vi "Plugin - Long Offset.vi"(11 "Message Queues in":T2) -> ()   [LabVIEW 2019]
uses:
  support/Copy of Message Queue/All Message Queues.ctl
  support/Copy of Message Queue/Message Cluster.ctl
  controls/WhieBackgroundHistogram.ctl
  Analysis/Global Tube Measurement.vi
  Acquisition/Acquisition.lvlib
  Analysis/Analysis.lvlib
  <vilib>/Analysis/NI_AALBase.lvlib
  <vilib>/ptbypt/NI_PtbyPt.lvlib
  support/Message Queue/Message Queue.lvlib
  support/Copy of Message Queue/Copy of Message Queue.lvlib
panel:
  out "Range(m)":dbl
  out "Ring Time (ms)":dbl format="%.2f"
  out "SSC Out(m)":dbl format="%0.4f"
  out "Offset Mean(m)":dbl format="%0.4f"
  out "Offset Std(m)":dbl format="%0.4f"
  in  "Stop":bool
  out "Time vs. Offset/Cor Offset":cluster{"Cor Offset":dbl, "Offset":dbl}(graph)
  out "Histogram Graph":T1
  out "T12":dbl(slide) scale=0.0..30.0
  out "T11":dbl(slide) scale=0.0..30.0
  out "T10":dbl(slide) scale=0.0..30.0
  out "T9":dbl(slide) scale=0.0..30.0
  out "T8":dbl(slide) scale=0.0..30.0
  out "T7":dbl(slide) scale=0.0..30.0
  out "T6":dbl(slide) scale=0.0..30.0
  out "T5":dbl(slide) scale=0.0..30.0
  out "T4":dbl(slide) scale=0.0..30.0
  out "T3":dbl(slide) scale=0.0..30.0
  out "T2":dbl(slide) scale=0.0..30.0
  out "T1":dbl(slide) scale=0.0..30.0
  out "Ring Time":waveform(dbl)(graph)
  out "Aquatrak RS232 Output":string
  in  "error in":errorcluster
  out "error out":errorcluster
  # "Calulating Long Offset"
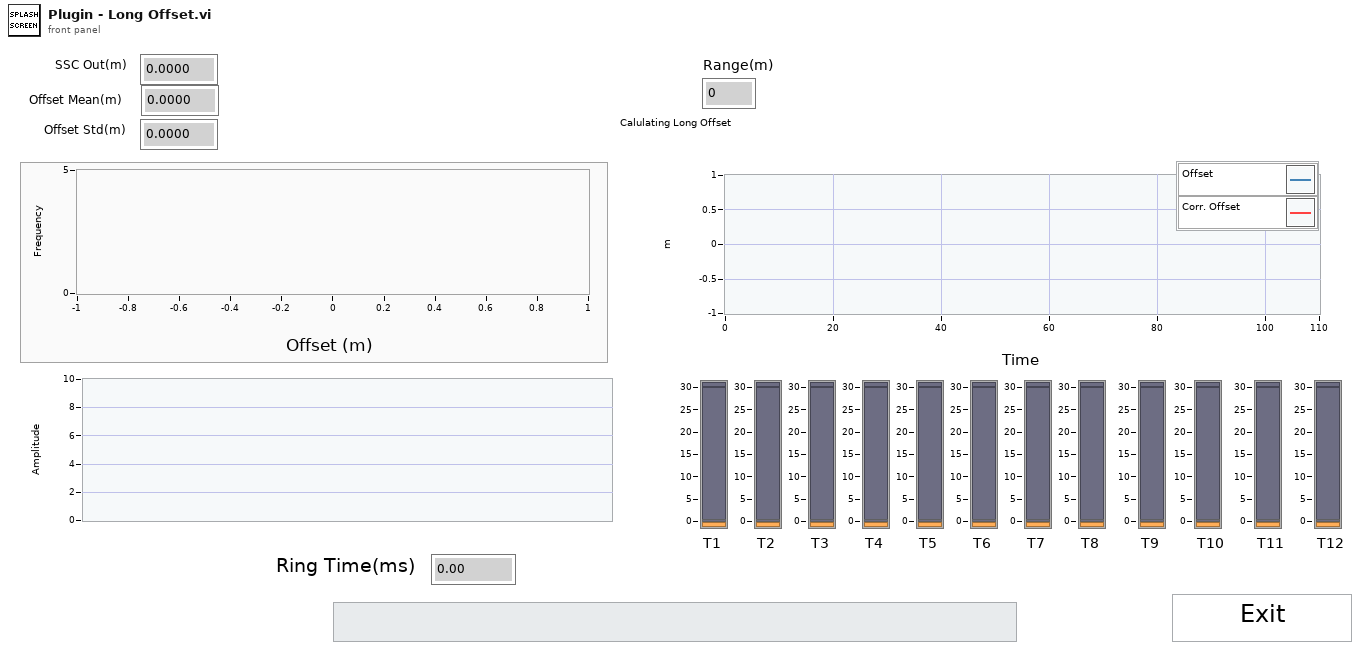
[diagram p1: front panel]
types:
  T1 = typedef "WhieBackgroundHistogram.ctl" = cluster{"X Values":dbl[], "Histogram: h(x)":i32[]}
  T2 = typedef "Copy of Message Queue.lvlib/All Message Queues.ctl" = cluster{"UI":refnum<queue>, "Acquisition":refnum<queue>, "Logging":refnum<queue>, "Analyze":refnum<queue>}
  T3 = cluster{"X Values":dbl[], "Histogram: h(x)":i32[]}
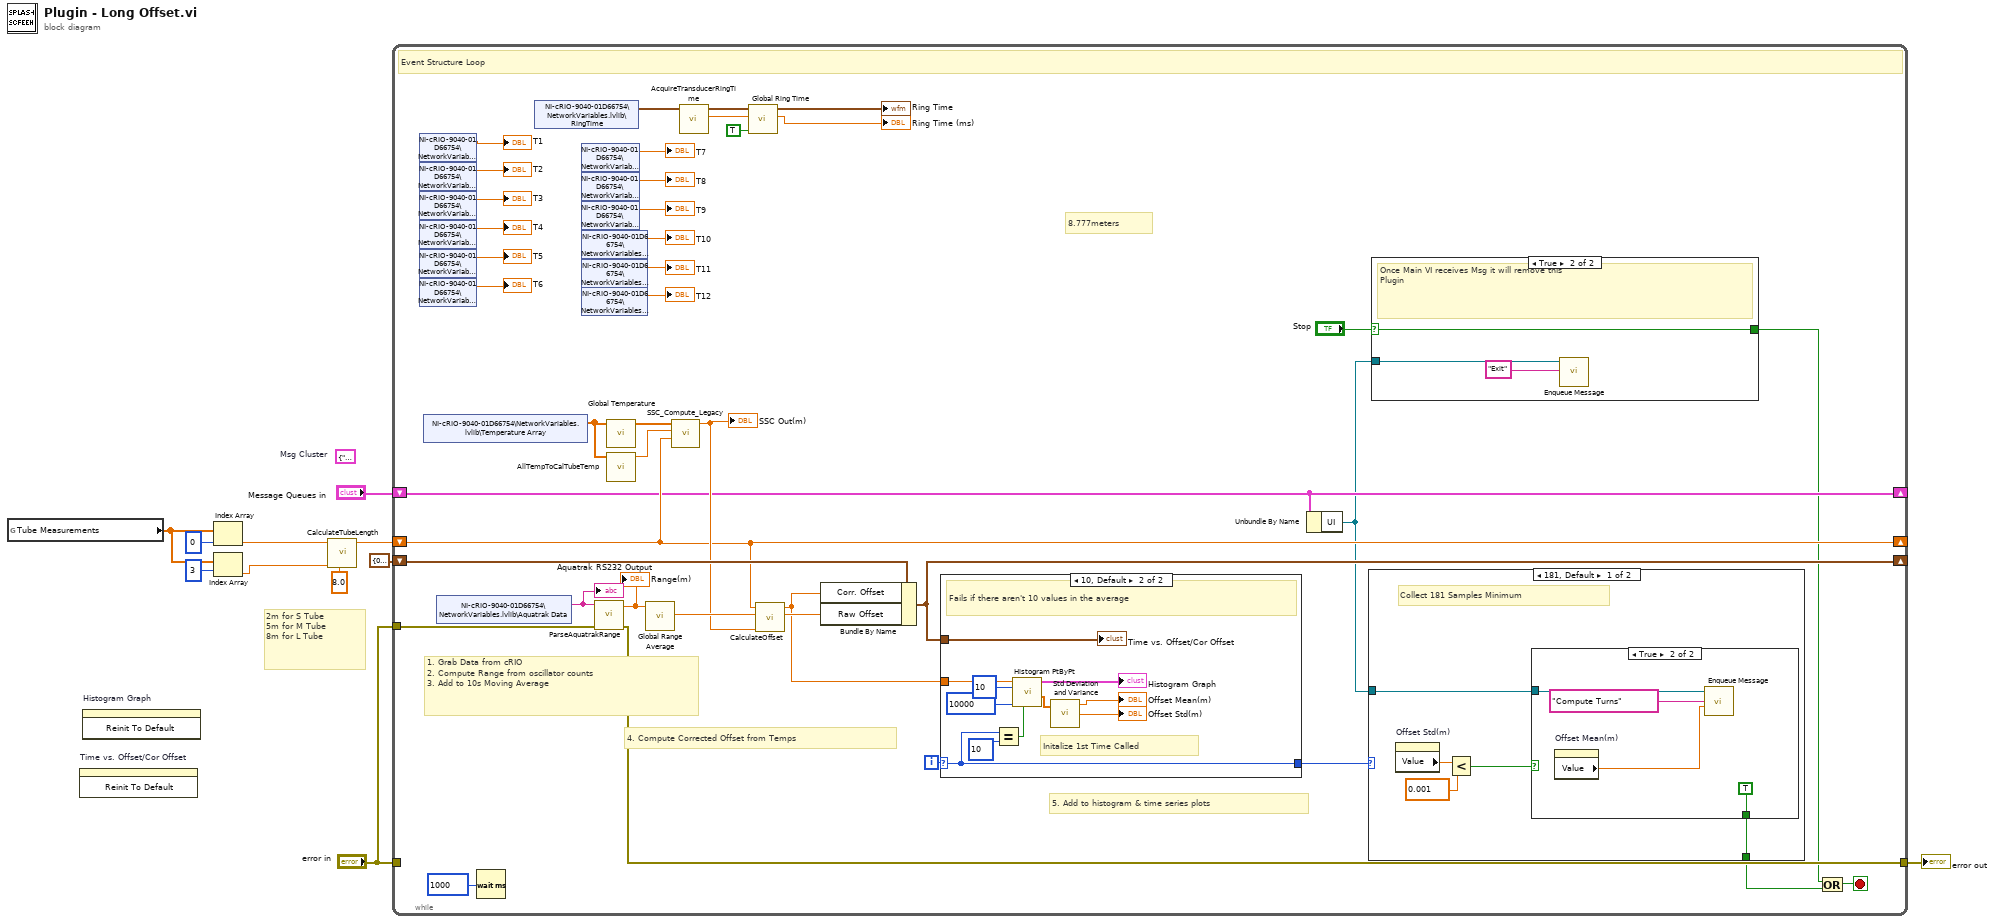
[diagram p0: block diagram]
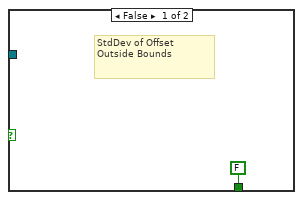
[diagram p3: hidden frame]
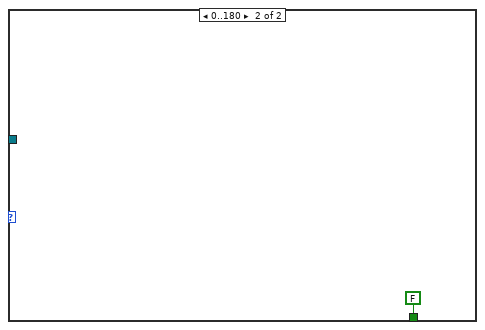
[diagram p4: hidden frame]
diagram:
  (unwired) cluster{"Msg":string, "Data":variant} {"Msg"="", "Data"=variant}  # Msg Cluster
  # "2m for S Tube\n5m for M Tube\n8m for L Tube"
  n1 = global read "Global Tube Measurement.vi" "Tube Measurements"() -> (w10:dbl[])
  n2 = invoke on="Time vs. Offset/Cor Offset" class="WFChart (strict)" method="Reinit To Default"() -> ()  [unwired: 3 in, 3 out]
  n3 = invoke on="Histogram Graph" class="XYGraph (strict)" method="Reinit To Default"() -> ()  [unwired: 3 in, 3 out]
  n4 = Index Array(array=w10, index=0) -> (element=w6:dbl)
  n5 = Index Array(array=w10, index=3) -> (element=w1:dbl)
  n6 = call "CalculateTubeLength.vi"("Range"=8.0, "Long Tube"=w1, "Collar"=w6) -> ("Tube Length"=w7:dbl)  [unwired: 8 in]
  n7 = while {
    shift-right: [w18] -> _
    shift-left: "Message Queues in" -> [w18]
    tunnel: "error in" -> [_]
    shift-right: [w20] -> _
    shift-left: cluster{"Raw Offset":dbl, "Corr. Offset":dbl} {"Raw Offset"=0.0, "Corr. Offset"=0.0} -> [w36]
    shift-right: [w21] -> _
    shift-left: w7 -> [w21]
    tunnel: [w25] -> w4
    tunnel: "error in" -> [w26]
    i -> [w22]
    stop <- w15 stop-if-true
    # "8.777meters"
    # "5. Add to histogram & time series plots"
    # "4. Compute Corrected Offset from Temps"
    # "1. Grab Data from cRIO\n2. Compute Range from oscillator counts \n3. Add to 10s Moving Average"
    # "Event Structure Loop"
    n8 = shared-variable "NI-cRIO-9040-01D66754\\NetworkVariables.lvlib\\T1"() -> (→"T1":dbl)  [unwired: 1 in, 1 out]
    n9 = shared-variable "NI-cRIO-9040-01D66754\\NetworkVariables.lvlib\\T2"() -> (→"T2":dbl)  [unwired: 1 in, 1 out]
    n10 = shared-variable "NI-cRIO-9040-01D66754\\NetworkVariables.lvlib\\T3"() -> (→"T3":dbl)  [unwired: 1 in, 1 out]
    n11 = shared-variable "NI-cRIO-9040-01D66754\\NetworkVariables.lvlib\\T4"() -> (→"T4":dbl)  [unwired: 1 in, 1 out]
    n12 = shared-variable "NI-cRIO-9040-01D66754\\NetworkVariables.lvlib\\T5"() -> (→"T5":dbl)  [unwired: 1 in, 1 out]
    n13 = shared-variable "NI-cRIO-9040-01D66754\\NetworkVariables.lvlib\\T6"() -> (→"T6":dbl)  [unwired: 1 in, 1 out]
    n14 = shared-variable "NI-cRIO-9040-01D66754\\NetworkVariables.lvlib\\Temperature Array"() -> (w34:dbl[])  [unwired: 1 in, 1 out]
    n15 = shared-variable "NI-cRIO-9040-01D66754\\NetworkVariables.lvlib\\Aquatrak Data"() -> (w35:string)  [unwired: 1 in, 1 out]
    "Aquatrak RS232 Output" <- w35
    n16 = Wait (ms)(milliseconds to wait=u32 1000) -> ()  [unwired: 1 out]
    n17 = shared-variable "NI-cRIO-9040-01D66754\\NetworkVariables.lvlib\\RingTime"() -> (w52:waveform(dbl)[])  [unwired: 1 in, 1 out]
    n18 = shared-variable "NI-cRIO-9040-01D66754\\NetworkVariables.lvlib\\T7"() -> (→"T7":dbl)  [unwired: 1 in, 1 out]
    n19 = shared-variable "NI-cRIO-9040-01D66754\\NetworkVariables.lvlib\\T8"() -> (→"T8":dbl)  [unwired: 1 in, 1 out]
    n20 = shared-variable "NI-cRIO-9040-01D66754\\NetworkVariables.lvlib\\T9"() -> (→"T9":dbl)  [unwired: 1 in, 1 out]
    n21 = shared-variable "NI-cRIO-9040-01D66754\\NetworkVariables.lvlib\\T10"() -> (→"T10":dbl)  [unwired: 1 in, 1 out]
    n22 = shared-variable "NI-cRIO-9040-01D66754\\NetworkVariables.lvlib\\T11"() -> (→"T11":dbl)  [unwired: 1 in, 1 out]
    n23 = shared-variable "NI-cRIO-9040-01D66754\\NetworkVariables.lvlib\\T12"() -> (→"T12":dbl)  [unwired: 1 in, 1 out]
    n24 = call "ParseAquatrakRange.vi"("error in"=w26, "Incoming String"=w35) -> ("error out"=w25:errorcluster, "Range(m)"=w38:dbl)  [unwired: 5 in, 3 out]
    "Range(m)" <- w38
    n25 = call "Global Temperature.vi"("Temp In"=w34) -> ("Temp Out"=w33:dbl[])  [unwired: 9 in, 1 out]
    n26 = call "AllTempToCalTubeTemp.vi"("All Temps"=w34) -> ("Cal Tube Temp"=w32:dbl)  [unwired: 10 in]
    n27 = call "Global Range Average.vi"("Range In"=w38) -> ("Average Range"=w39:dbl)  [unwired: 9 in, 1 out]
    n28 = call "SSC_Compute_Legacy.vi"("Tube Length"=w21, "Cal Tube Temp"=w32, "Sound Tube Temp"=w33) -> ("SSC Out(m)"=w31:dbl)  [unwired: 8 in]
    "SSC Out(m)" <- w31
    n29 = call "AcquireTransducerRingTime.vi"("Ring Time Wavefrom Array"=w52) -> ("Ring Time (ms)"=w29:dbl, "Ring Time Wavefrom"=w30:waveform(dbl))  [unwired: 8 in, 1 out]
    n30 = call "Global Ring Time.vi"("Ring Time Plot In"=w30, "Ring Time (ms) In"=w29, "Set Data?"=TRUE) -> ("Ring Time Plot Out"=→"Ring Time":waveform(dbl), "Ring Time (ms) Out"=→"Ring Time (ms)":dbl)  [unwired: 6 in]
    n31 = call "CalculateOffset.vi"("SSC"=w31, "Range"=w39, "Tube Length"=w21) -> ("Raw Offset Value"=w37:dbl, "Offset Value"=w23:dbl)  [unwired: 7 in]
    n32 = Bundle By Name(cluster=w36, "Corr. Offset"=w23, "Raw Offset"=w37) -> (w20:cluster{"Raw Offset":dbl, "Corr. Offset":dbl})
    n33 = case shown="10, Default" w22 {
      selector: w22 -> [w68 w70]
      tunnel: w23 -> [_ w76]
      tunnel: w20 -> [_ w75]
      tunnel: [w68 w70] -> w19
      frame 0..9 {
        # "Fails if there aren't 10 values in the average"
      }
      frame 10, Default {
        # "Initalize 1st Time Called"
        # "Fails if there aren't 10 values in the average"
        n34 = Equal?(x=w70, y=10 ("intervals")) -> (x = y?=w71:bool)
        n35 = call <vilib>:"Histogram PtByPt.vi"("initialize"=w71, "sample length"=10000, "intervals"=10, "x"=w76) -> ("X Values"=w77:dbl[], "Histogram Graph"=→"Histogram Graph":T3)  [unwired: 4 in, 2 out]
        n36 = call <vilib>:"Std Deviation and Variance.vi"("X"=w77) -> ("mean"=→"Offset Mean(m)":dbl, "standard deviation"=→"Offset Std(m)":dbl)  [unwired: 1 in, 1 out]
        "Time vs. Offset/Cor Offset" <- w75
      }
    }
    n37 = Unbundle By Name(w18) -> ("UI"=w16:refnum<queue>)
    n38 = case shown="181, Default" w19 {
      tunnel: [w57 FALSE] -> w13
      tunnel: w16 -> [w61 _]
      frame 181, Default {
        # "Collect 181 Samples Minimum"
        n39 = property on="Offset Std(m)" class="DigNum (strict)"() -> ("Value"=w60:dbl)  [unwired: 2 in, 2 out]
        n40 = Less?(x=w60, y=0.001) -> (x < y?=w59:bool)
        n41 = case shown="True" w59 {
          tunnel: w61 -> [_ w65]
          tunnel: [FALSE TRUE] -> w57
          frame False {
            # "StdDev of Offset\nOutside Bounds"
          }
          frame True {
            n42 = property on="Offset Mean(m)" class="DigNum (strict)"() -> ("Value"=w64:dbl)  [unwired: 2 in, 2 out]
            n43 = call "Enqueue Message.vi"("Message Data"=w64, "Message"="Compute Turns", "Message Queue"=w65) -> ()  [unwired: 7 in, 2 out]
          }
        }
      }
      frame 0..180 {
      }
    }
    n44 = case shown="True" "Stop" {
      selector: "Stop" -> [w53 w54]
      tunnel: w16 -> [_ w55]
      tunnel: [w53 w54] -> w14
      frame False {
      }
      frame True {
        # "Once Main VI receives Msg it will remove this \nPlugin"
        n45 = call "Enqueue Message.vi"("Message"="Exit", "Message Queue"=w55) -> ()  [unwired: 8 in, 2 out]
      }
    }
    n46 = Or(x=w14, y=w13) -> (x .or. y?=w15:bool)
  }
  "error out" <- w4
